vi "Traverse FP for Control Refs.vi"(8 "error in (no error)":errorcluster, 11 "VI Ref":refnum<vi>) -> (0 "error out":errorcluster, 2 "Control Refs":refnum<vi>[](array[refnum]), 3 "VI Ref out":refnum<vi>)   [LabVIEW 2020, in "VI Properties Editor.lvlib"]
doc: "Traverses the front panel of the VI identified by <B>VI Ref</B> for all control references."
uses:
  VI Properties Editor.lvlib
  <vilib>/Utility/traverseref.llb/TRef TravTarget.ctl
  <vilib>/Utility/traverseref.llb/VI Scripting - Traverse.lvlib
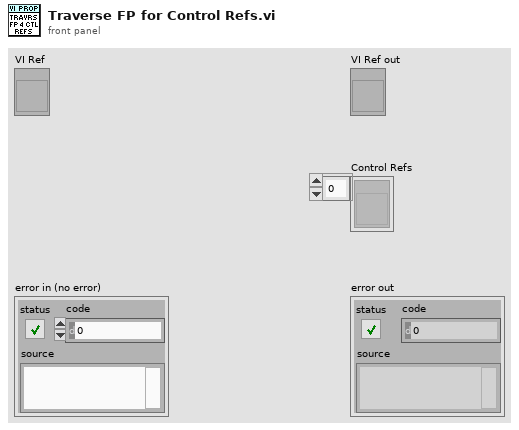
[diagram p1: front panel]
types:
  T1 = typedef "TRef TravTarget.ctl" = enum16{"FP", "BD", "Other"}
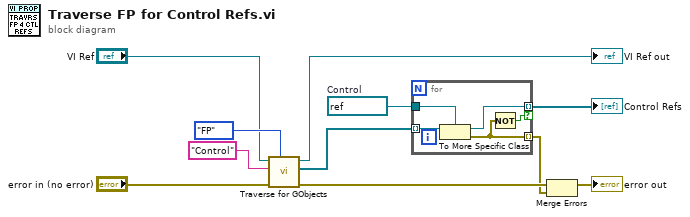
[diagram p0: block diagram]
diagram:
  w2 = refnum<vi> refnum  # Control
  n1 = call <vilib>:"Traverse for GObjects.vi"("Traverse Target"=TRef_TravTarget."FP", "error in (no error)"="error in (no error)", "Class Name"="Control", "VI Refnum"="VI Ref") -> ("error out"=w7:errorcluster, "References"=w5:refnum<vi>[], "dup VI Refnum"=→"VI Ref out":refnum<vi>)  [unwired: 4 in, 1 out]
  n2 = for {
    tunnel: w5 -> [w16] mode=indexing
    tunnel: [w15] -> w1 mode=indexing if=w14
    tunnel: [w13] -> w3 mode=indexing
    tunnel: w2 -> [w12]
    n3 = To More Specific Class(target class=w12, reference=w16) -> (specific class reference=w15:refnum<vi>, error out=w13:errorcluster)  [unwired: 1 in]
    n4 = Not(x=w13) -> (.not. x?=w14:bool)
  }
  "Control Refs" <- w1
  n5 = Merge Errors(w7, w3) -> (→"error out":errorcluster)
